vi "FilterAndStats.vi"(0 "TempIn":dbl=25.0, 1 "Reset":bool) -> (2 "MovAvg":dbl, 3 "MinOut":dbl, 4 "MaxOut":dbl)   [LabVIEW 2025]
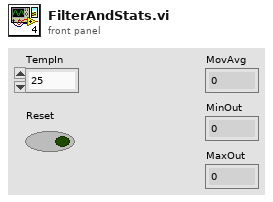
[diagram p1: front panel]
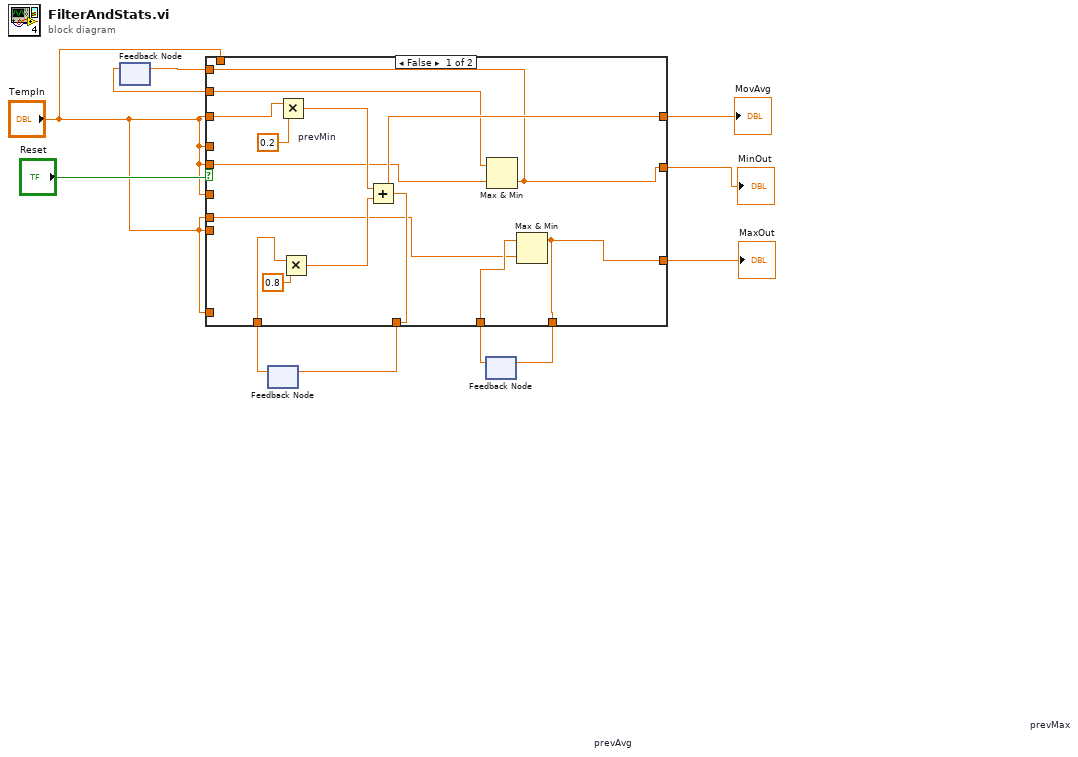
[diagram p0: block diagram]
diagram:
  n1 = feedback #1 "prevMin"() -> (w6:dbl)  [unwired: 1 in]
  n2 = feedback #2 "prevAvg"() -> (w8:dbl)  [unwired: 1 in]
  n3 = feedback #3 "prevMax"() -> (w4:dbl)  [unwired: 1 in]
  n4 = case shown="False" "Reset" {
    tunnel: "TempIn" -> [w22 w30]
    tunnel: [w18 w30] -> w10
    tunnel: "TempIn" -> [_ w25]
    tunnel: "TempIn" -> [_ w29]
    tunnel: [w12 w29] -> w9
    tunnel: w8 -> [w23 _]
    tunnel: [w18 w27] -> w7
    tunnel: w6 -> [w17 _]
    tunnel: "TempIn" -> [w16 _]
    tunnel: [w13 w28] -> w5
    tunnel: w4 -> [w15 _]
    tunnel: "TempIn" -> [w14 _]
    tunnel: [w12 w26] -> w3
    tunnel: "TempIn" -> [_ w28]
    tunnel: "TempIn" -> [_ w27]
    tunnel: "TempIn" -> [_ w26]
    tunnel: [w13 w25] -> w1
    frame False {
      n5 = Multiply(x=w22, y=0.2) -> (x*y=w20:dbl)
      n6 = Multiply(x=w23, y=0.8) -> (x*y=w19:dbl)
      n7 = Add(x=w20, y=w19) -> (x+y=w18:dbl)
      n8 = Max & Min(x=w17, y=w16) -> (min(x,y)=w13:dbl)  [unwired: 1 out]
      n9 = Max & Min(x=w15, y=w14) -> (max(x,y)=w12:dbl)  [unwired: 1 out]
    }
    frame True {
    }
  }
  "MovAvg" <- w10
  "MinOut" <- w1
  "MaxOut" <- w9
  n10 = feedback-in #1(w5) -> ()
  n11 = feedback-in #2(w7) -> ()
  n12 = feedback-in #3(w3) -> ()
